vi "Error.vi"(8 "error in (no error)":errorcluster, 10 "error":errorcluster, 11 "Error Manager in":refnum<class "Error Manager.lvclass">) -> (0 "error out":errorcluster, 3 "Error Manager out":refnum<class "Error Manager.lvclass">)   [LabVIEW 2024, in "Error Manager.lvlib" / "Error Manager.lvclass"]
uses:
  Error Manager.lvclass
  Error Manager.lvclass/Error Manager.ctl
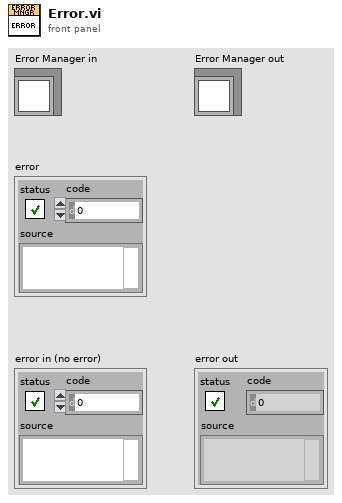
[diagram p1: front panel]
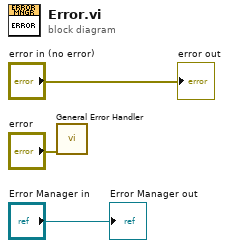
[diagram p0: block diagram]
diagram:
  n1 = call <vilib>:"General Error Handler.vi"("error in (no error)"="error") -> ()  [unwired: 10 in, 5 out]
  "error out" <- "error in (no error)"
  "Error Manager out" <- "Error Manager in"
